vi "send_analysis_data_to_AnalysisObj.vi"(0 "SessionID":string, 5 "plotname":string, 7 "time in":dbl, 9 "value":dbl, 11 "error in (no error)":errorcluster, 12 "flag in (0,1)":string="0") -> (15 "error out":errorcluster)   [LabVIEW 2018]
doc: "sendds the data to the AnalysisSession (SessionID) and stores them in the AnalysisDataArray"
uses:
  Classes/Analysis/Analysis.lvclass
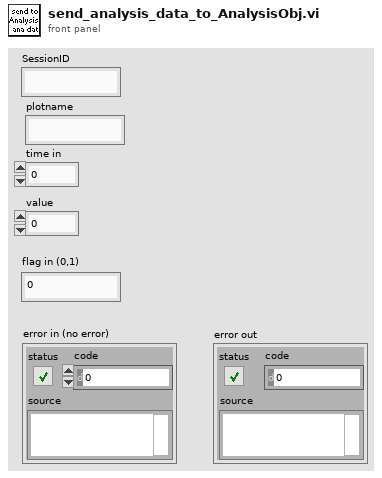
[diagram p1: front panel]
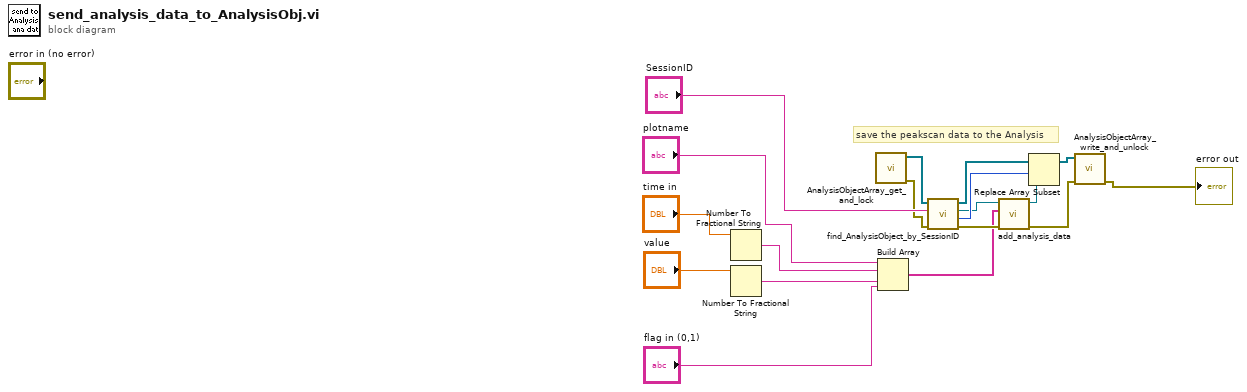
[diagram p0: block diagram]
diagram:
  # "save the peakscan data to the Analysis"
  n1 = Number To Fractional String(number="time in") -> (F-format string=w16:string)  [unwired: 3 in]
  n2 = Number To Fractional String(number="value") -> (F-format string=w17:string)  [unwired: 3 in]
  n3 = call "AnalysisObjectArray_get_and_lock.vi"() -> ("error out"=w6:errorcluster, "AnalysisObjects"=w3:refnum<class "Analysis.lvclass">[])  [unwired: 10 in]
  n4 = Build Array("plotname", w16, w17, "flag in (0,1)") -> (w2:string[])
  n5 = call "find_AnalysisObject_by_SessionID.vi"("error in (no error)"=w6, "SessionID"="SessionID", "AnalysisObjects in"=w3) -> ("error out"=w5:errorcluster, "index of found"=w9:i32, "found AnalyisObject"=w4:refnum<class "Analysis.lvclass">, "AnalysisObjects out"=w7:refnum<class "Analysis.lvclass">[])  [unwired: 5 in]
  n6 = call-dynamic "add_analysis_data.vi"("error in (no error)"=w5, "single analysis data"=w2, "Analysis in"=w4) -> ("error out"=w11:errorcluster, "Analysis out"=w8:refnum<class "Analysis.lvclass">)  [unwired: 7 in]
  n7 = Replace Array Subset(array=w7, new element=w8, index=w9) -> (w10:refnum<class "Analysis.lvclass">[])
  n8 = call "AnalysisObjectArray_write_and_unlock.vi"("error in (no error)"=w11, "AnalysisObjects"=w10) -> ("error out"=→"error out":errorcluster)  [unwired: 9 in]
